vi "FlushQueue.vi"(8 "ErrorArray":errorcluster[](array[cluster])) -> (0 "ErrorArray Out":errorcluster[](array[cluster]))   [LabVIEW 2018, in "Test.lvclass"]
uses:
  Test.lvclass
  <userlib>/NIST/NISTErrorLib/NISTErrorLib.lvlib
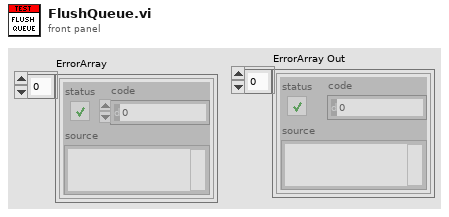
[diagram p1: front panel]
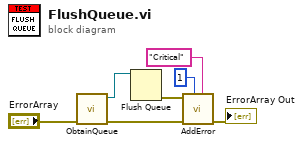
[diagram p0: block diagram]
diagram:
  n1 = call "ObtainQueue.vi"("ErrorArray"="ErrorArray") -> ("ErrorArray."=w3:errorcluster[], "TstQue"=w6:refnum<queue>)  [unwired: 9 in]
  n2 = Flush Queue(queue=w6) -> (error out=w5:errorcluster)  [unwired: 1 in, 2 out]
  n3 = call <userlib>:"AddError.vi"("Severity"="Critical", "Priority"=u8 1, "ErrorArray In"=w3, "error in (no error)"=w5) -> ("ErrorArray Out"=→"ErrorArray Out":errorcluster[])  [unwired: 6 in, 1 out]
